vi "Initialize Channel Selector.vi"(8 "error in (no error)":errorcluster, 11 "Phasor Data Concentrator in":refnum<class "Phasor Data Concentrator.lvclass">) -> (0 "error out":errorcluster, 3 "Phasor Data Concentrator out":refnum<class "Phasor Data Concentrator.lvclass">)   [LabVIEW 2013, in "PMU Recorder Light.lvlib" / "Phasor Data Concentrator.lvclass"]
uses:
  Phasor Data Concentrator.lvclass
  Phasor Data Concentrator.lvclass/Phasor Data Concentrator.ctl
  PMU Recorder Light.lvlib
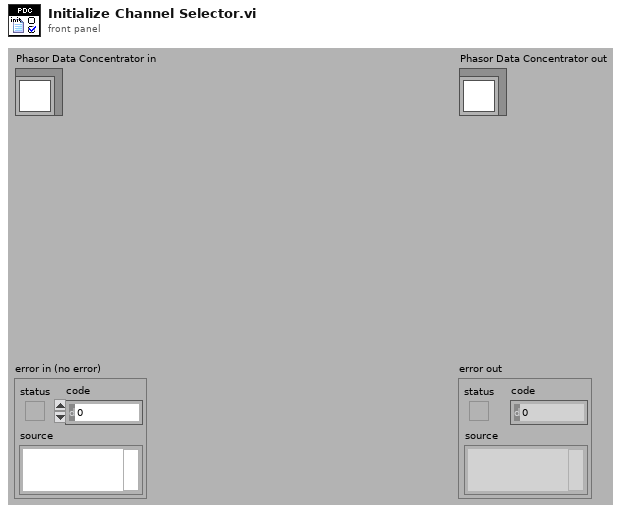
[diagram p1: front panel]
types:
  T1 = cluster{"Phasor":string[], "Analog":string[], "Digital":string[]}
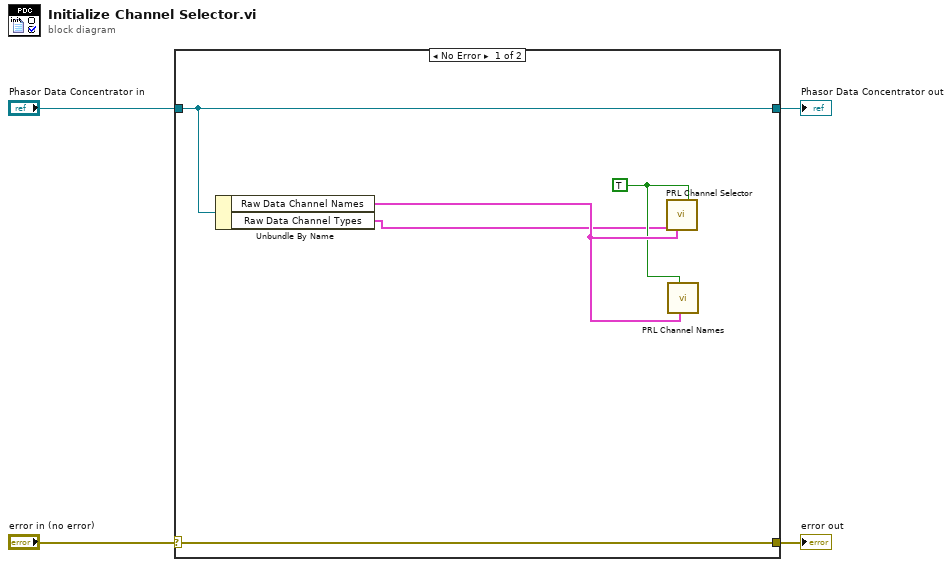
[diagram p0: block diagram]
diagram:
  n1 = case shown="No Error" "error in (no error)" {
    selector: "error in (no error)" -> [w9 w11]
    tunnel: [w9 w11] -> w3
    tunnel: [w8 w10] -> w1
    tunnel: "Phasor Data Concentrator in" -> [w8 w10]
    frame No Error {
      w6 = TRUE ("Initialize?")
      n2 = Unbundle By Name(w8) -> ("Raw Data Channel Names"=w7:T1, "Raw Data Channel Types"=w5:cluster{"Phasor":u8[], "Analog":u8[]})
      n3 = call "PRL Channel Selector.vi"("Initialize?"=w6, "Signal Types"=w5, "Signal Names In"=w7) -> ()  [unwired: 9 in, 4 out]
      n4 = call "PRL Channel Names.vi"("Details"=w7, "Initialize?"=w6) -> ()  [unwired: 7 in, 3 out]
    }
    frame Error {
    }
  }
  "error out" <- w3
  "Phasor Data Concentrator out" <- w1
